vi "Create Find and Replace Array for Word.vi"(8 "error in":errorcluster, 10 "Mathcad Output":T1, 11 "DesignRequest":T2) -> (0 "error out":errorcluster, 3 "Find-Replace":cluster{"Find":string, "Replace":string}[](array[cluster]))   [LabVIEW 2015]
uses:
  Variable cluster.ctl
  Design Request.ctl
panel:
  out "appended array":T1
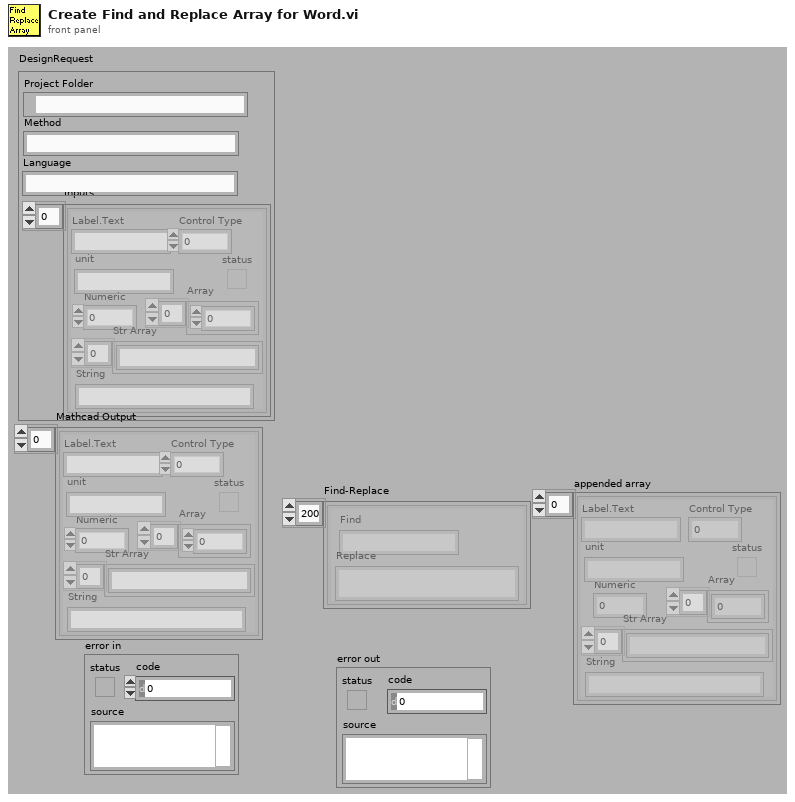
[diagram p1: front panel]
types:
  T1 = typedef "Variable cluster.ctl" = cluster{"Label.Text":string, "Control Type":u32, "Numeric":dbl, "Array":dbl[], "status":bool, "Str Array":string[], "String":string, "unit":string}[]
  T2 = typedef "Design Request.ctl" = cluster{"Project Folder":path, "Method":string, "Inputs":T1, "Language":string}
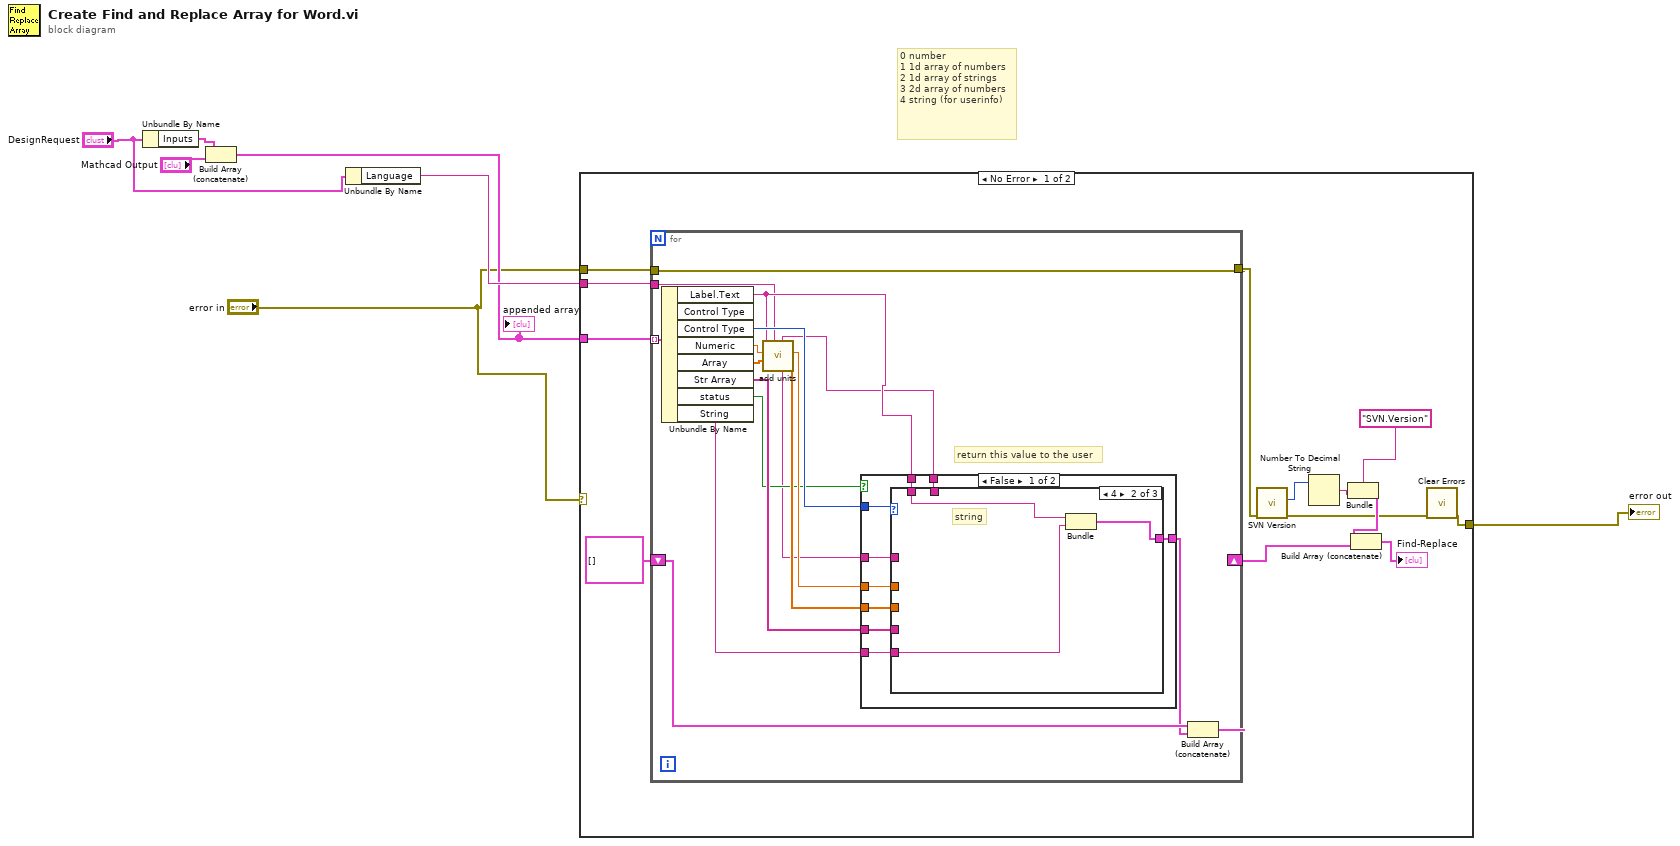
[diagram p0: block diagram]
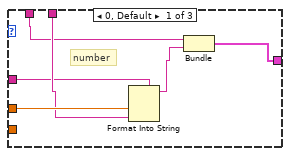
[diagram p2: hidden frame]
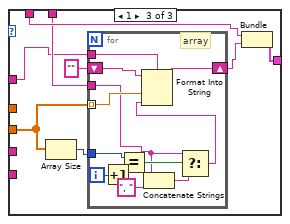
[diagram p3: hidden frame]
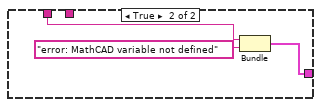
[diagram p4: hidden frame]
diagram:
  # "0\tnumber\n1\t1d array of numbers\n2\t1d array of strings\n3\t2d array of numbers\n4 string (for userinfo)"
  n1 = Unbundle By Name("DesignRequest") -> ("Inputs"=w3:T1)
  n2 = Build Array (concatenate)(w3, "Mathcad Output") -> (w4:T1)
  "appended array" <- w4
  n3 = Unbundle By Name("DesignRequest") -> ("Language"=w7:string)
  n4 = case shown="No Error" "error in" {
    selector: "error in" -> [_ w79]
    tunnel: w7 -> [w20 _]
    tunnel: [w15 w79] -> w6
    tunnel: w4 -> [w11 _]
    tunnel: "error in" -> [w10 _]
    frame No Error {
      n5 = for {
        tunnel: w10 -> [w35]
        tunnel: [w35] -> w8
        tunnel: w11 -> [w37] mode=indexing
        tunnel: w20 -> [w22]
        shift-right: [w25] -> w19
        shift-left: cluster{"Label.Text":string, "string":string}[] [] -> [w26]
        # "return this value to the user"
        n6 = Unbundle By Name(w37) -> ("Label.Text"=w28:string, "Control Type"=w36:u32, "Numeric"=w32:dbl, "Array"=w33:dbl[], "Str Array"=w34:string[], "status"=w29:bool, "String"=w23:string)  [unwired: 1 out]
        n7 = call "add units.vi"("Language"=w22, "Array"=w33, "Numeric"=w32, "Label Text"=w28) -> ("Converted Array"=w31:dbl[], "Converted Numeric"=w30:dbl, "format string"=w24:string, "unit"=w27:string)  [unwired: 3 in, 1 out]
        n8 = case shown="False" w29 {
          tunnel: w36 -> [w46 _]
          tunnel: w30 -> [w45 _]
          tunnel: w31 -> [w44 _]
          tunnel: w27 -> [w43 _]
          tunnel: [w42 w77] -> w21
          tunnel: w34 -> [w41 _]
          tunnel: w28 -> [w40 w78]
          tunnel: w24 -> [w39 _]
          tunnel: w23 -> [w38 _]
          frame False {
            n9 = case shown="4" w46 {
              tunnel: [w48 w54 w61] -> w42
              tunnel: w45 -> [w52 _ _]
              tunnel: w44 -> [_ _ w62]
              tunnel: w43 -> [w51 _ w58]
              tunnel: w41 -> [_ _ _]
              tunnel: w40 -> [w50 w55 w60]
              tunnel: w39 -> [w47 _ w56]
              tunnel: w38 -> [_ w53 _]
              frame 0, Default {
                # "number"
                n10 = Format Into String(format string=w47, w52, w51) -> (resulting string=w49:string)  [unwired: 2 in, 1 out]
                n11 = Bundle("Label.Text"=w50, w49) -> (w48:cluster{"Label.Text":string, string})  [unwired: 1 in]
              }
              frame 4 {
                # "string"
                n12 = Bundle("Label.Text"=w55, "String"=w53) -> (w54:cluster{"Label.Text":string, "String":string})  [unwired: 1 in]
              }
              frame 1 {
                n13 = Array Size(array=w62) -> (size(s)=w63:i32)
                n14 = for {
                  shift-right: [w75] -> w59
                  shift-left: "" -> [w69]
                  tunnel: w62 -> [w70] mode=indexing
                  tunnel: w63 -> [w72]
                  tunnel: w58 -> [w65]
                  tunnel: w56 -> [w68]
                  i -> [w74]
                  # "array"
                  n15 = Increment(x=w74) -> (x+1=w71:i32)
                  n16 = Equal?(x=w72, y=w71) -> (x = y?=w73:bool)
                  n17 = Concatenate Strings(w65, ", " ("string")) -> (w67:string)
                  n18 = Select(t=w65, s=w73, f=w67) -> (s? t:f=w64:string)
                  n19 = Format Into String(format string=w68, initial string=w69, w70, w64) -> (resulting string=w75:string)  [unwired: 1 in, 1 out]
                }
                n20 = Bundle("Label.Text"=w60, w59) -> (w61:cluster{"Label.Text":string, string})  [unwired: 1 in]
              }
            }
          }
          frame True {
            n21 = Bundle("Label.Text"=w78, "string"="error: MathCAD variable not defined") -> (w77:cluster{"Label.Text":string, "string":string})  [unwired: 1 in]
          }
        }
        n22 = Build Array (concatenate)(w26, w21) -> (w25:cluster{"Label.Text":string, "string":string}[])
      }
      n23 = call "SVN Version.vi"("error in (no error)"=w8) -> ("error out"=w16:errorcluster, "Revision"=w13:i32)  [unwired: 6 in, 3 out]
      n24 = Number To Decimal String(number=w13) -> (decimal integer string=w12:string)  [unwired: 1 in]
      n25 = Bundle("Version string"="SVN.Version", w12) -> (w18:cluster{"Version string":string, string})  [unwired: 1 in]
      n26 = Build Array (concatenate)(w18, w19) -> (→"Find-Replace":cluster{"Label.Text":string, "string":string}[])
      n27 = call <vilib>:"Clear Errors.vi"("error in (no error)"=w16) -> ("error out"=w15:errorcluster)  [unwired: 5 in, 1 out]
    }
    frame Error {
    }
  }
  "error out" <- w6
